vi "GetDataRealImage.vi"(11 "input":string) -> (2 "imag":dbl, 3 "real":dbl)   [LabVIEW 2012]
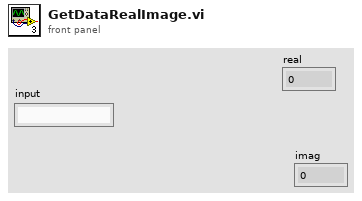
[diagram p1: front panel]
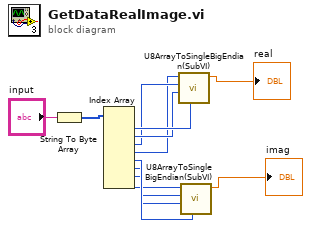
[diagram p0: block diagram]
diagram:
  n1 = String To Byte Array(string="input") -> (unsigned byte array=w11:u8[])
  n2 = Index Array(array=w11) -> (element #1=w10:u8, element #2=w9:u8, element #3=w8:u8, element #4=w7:u8, element #5=w6:u8, element #6=w5:u8, element #7=w4:u8, element #8=w3:u8)  [unwired: 8 in]
  n3 = call "U8ArrayToSingleBigEndian(SubVI).vi"("Numeric 5"=w10, "Numeric 4"=w9, "Numeric 3"=w8, "Numeric in"=w7) -> ("Numeric 8"=→"real":sgl)  [unwired: 7 in]
  n4 = call "U8ArrayToSingleBigEndian(SubVI).vi"("Numeric 5"=w6, "Numeric 4"=w5, "Numeric 3"=w4, "Numeric in"=w3) -> ("Numeric 8"=→"imag":sgl)  [unwired: 7 in]
